vi "DBGet.vi"() -> ()   [LabVIEW 2018]
uses:
  lib/Snap7.lvlib
panel:
  out "?":string
  out "Size Get":i32
  out "Running":bool
  out "Status":string="No Error"
  in  "DB Number":i32=1
  out "Data":u8[](array[numeric])
  in  "?":bool
  in  "Slot":i32=2
  in  "Rack":i32
  in  "Address IP":string="192.168.1.12"
  # "DB Get"
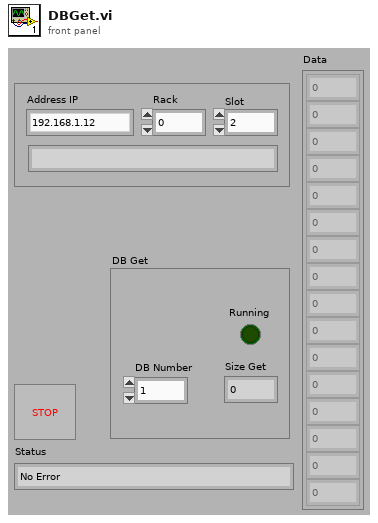
[diagram p1: front panel]
types:
  T1 = enum16{"big-endian, network order", "native, host order", "little-endian"}
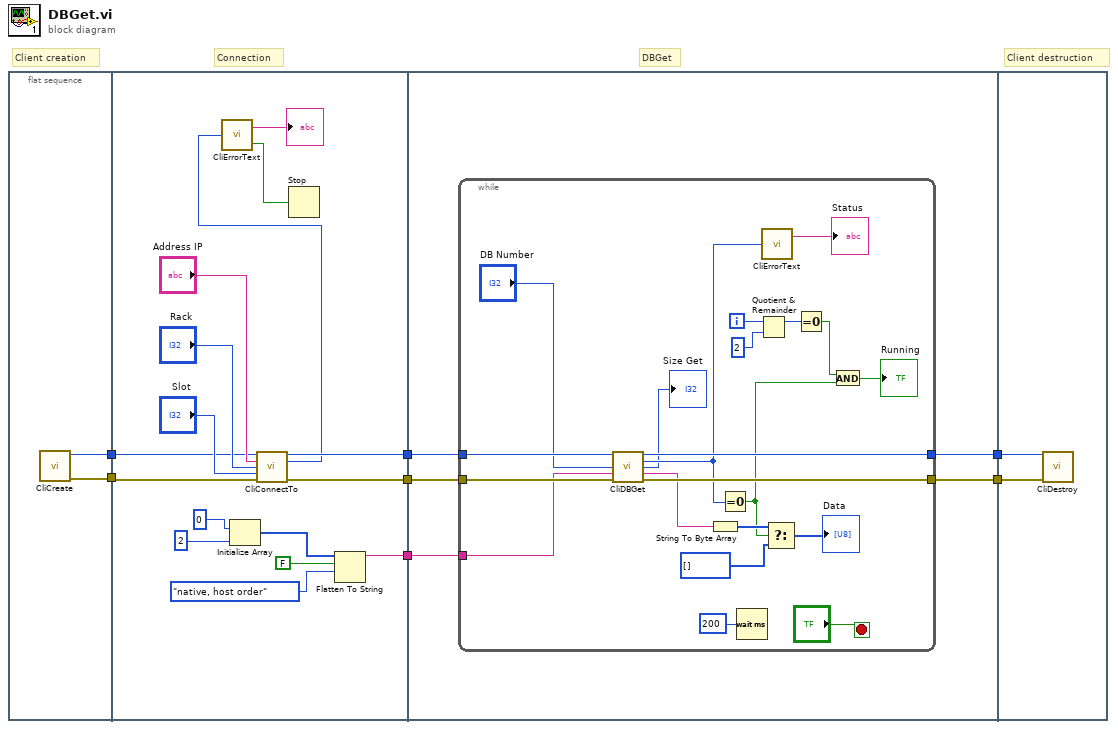
[diagram p0: block diagram]
diagram:
  # "Client destruction"
  # "DBGet"
  # "Connection"
  # "Client creation"
  n1 = flat-sequence {
    tunnel: [w9] -> w4
    tunnel: [w8] -> w3
    tunnel: [w20] -> w7
    tunnel: [w13] -> w6
    tunnel: [w19] -> w5
    tunnel: w4 -> [w15]
    tunnel: w3 -> [w14]
    tunnel: w7 -> [w30]
    tunnel: w6 -> [w29]
    tunnel: w5 -> [w28]
    tunnel: [w27] -> w2
    tunnel: [w26] -> w1
    tunnel: w2 -> [w53]
    tunnel: w1 -> [w52]
    frame #0 {
      n2 = call "CliCreate.vi"() -> ("ref out"=w9:u64, "error out"=w8:errorcluster)  [unwired: 14 in]
    }
    frame #1 {
      n3 = Initialize Array(u8 0, 2) -> (w23:u8[])
      n4 = call "CliConnectTo.vi"("ref in"=w15, "Address"="Address IP", "Rack"="Rack", "Slot"="Slot", "error in (no error)"=w14) -> ("ref out"=w13:u64, "Result"=w11:i32, "error out"=w20:errorcluster)  [unwired: 8 in]
      n5 = call "CliErrorText.vi"("ErrNo"=w11) -> ("Error"=w12:bool, "ErrMessage"=→"?":string)
      n6 = Stop(stop? (T)=w12) -> ()
      n7 = Flatten To String(anything=w23, prepend array or string size? (T)=FALSE, byte order (0:big-endian, network order)=T1."native, host order") -> (data string=w19:string)  [unwired: 1 in, 2 out]
    }
    frame #2 {
      n8 = while {
        tunnel: w30 -> [w49]
        tunnel: w29 -> [w48]
        tunnel: w28 -> [w35]
        tunnel: [w43] -> w27
        tunnel: [w42] -> w26
        i -> [w41]
        stop <- "?" stop-if-true
        n9 = call "CliDBGet.vi"("ref in"=w48, "DB Number"="DB Number", "data in"=w35, "error in (no error)"=w49) -> ("ref out"=w43:u64, "Result"=w33:i32, "SizeGet"=→"Size Get":i32, "data out"=w34:string, "error out"=w42:errorcluster)  [unwired: 7 in]
        n10 = String To Byte Array(string=w34) -> (unsigned byte array=w46:u8[])
        n11 = Equal To 0?(x=w33) -> (x = 0?=w36:bool)
        n12 = Wait (ms)(milliseconds to wait=u32 200 ("Loop Delay (ms)")) -> ()  [unwired: 1 out]
        n13 = Quotient & Remainder(x=w41, y=2) -> (x-y*floor(x/y)=w39:i32)  [unwired: 1 out]
        n14 = call "CliErrorText.vi"("ErrNo"=w33) -> ("ErrMessage"=→"Status":string)  [unwired: 1 out]
        n15 = Select(t=w46, s=w36, f=u8[] []) -> (s? t:f=→"Data":u8[])
        n16 = Equal To 0?(x=w39) -> (x = 0?=w38:bool)
        n17 = And(x=w38, y=w36) -> (x .and. y?=→"Running":bool)
      }
    }
    frame #3 {
      n18 = call "CliDestroy.vi"("ref in"=w53, "error in (no error)"=w52) -> ()  [unwired: 13 in, 1 out]
    }
  }
